vi "Open New WorkSheet.vi"(2 "error in (no error)":errorcluster, 4 "Excel._Workbook":refnum<k7>) -> (0 "error out":errorcluster, 1 "Excel._Worksheet":refnum<k7>)   [LabVIEW 2012]
doc: "Opens a Worksheet by name. Takes a Application Refnum as input. If the name is not connected or its string length is zero then it opens the first worksheet."
panel:
  in  "Excel._Worksheet":refnum<k7>
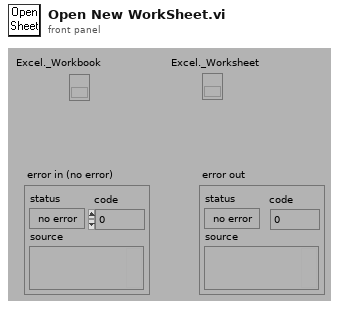
[diagram p1: front panel]
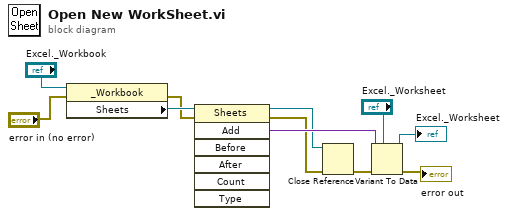
[diagram p0: block diagram]
diagram:
  n1 = property class="_Workbook"(reference="Excel._Workbook", error in="error in (no error)") -> (error out=w8:errorcluster, "Sheets"=w9:refnum<k7>)  [unwired: 1 out]
  n2 = invoke class="Sheets" method="Add"(reference=w9, error in=w8) -> (reference out=w3:refnum<k7>, error out=w2:errorcluster, "Add"=w7:variant)  [unwired: 5 in, 4 out]
  n3 = Close Reference(reference=w3, error in (no error)=w2) -> (error out=w1:errorcluster)
  n4 = Variant To Data(error in=w1, type="Excel._Worksheet", Variant=w7) -> (data=→"Excel._Worksheet":refnum<k7>, error out=→"error out":errorcluster)
